vi "Aufschaltung CalGas Span Name.vi"() -> (3 "Span Name":T1)   [LabVIEW 2020, in "Linearisierung v2.lvlib" / "SpanEinstellungen.lvlib"]
uses:
  SpanEinstellungen.lvlib
  Visualisierungs Elemente/String - Eingabefeld.ctl
  Seiten/CalGas Aufschaltung/FGV CalGas Aktionen.ctl
  Sprachverwaltung/FGV Aktion Tabelle zerlegen.ctl
  Seiten/CalGas Aufschaltung/CalGas Aufschaltung.lvlib
  Sprachverwaltung/Sprachverwaltung.lvlib
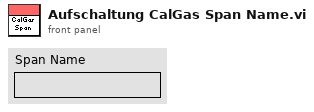
[diagram p1: front panel]
types:
  T1 = typedef "String - Eingabefeld.ctl" = string
  T2 = typedef "Sprachverwaltung.lvlib/FGV Aktion Tabelle zerlegen.ctl" = enum16{"laden", "vereinzeln", "speichern"}
  T3 = typedef "CalGas Aufschaltung.lvlib/FGV CalGas Aktionen.ctl" = enum16{"lesen", "Analysator Auswahl", "Def.CalGas", "Aufschaltung CalGas", "laden", "speichern", "KAL extrahieren"}
  T4 = typedef "CalGas Aufschaltung.lvlib/Aufschaltung CalGas.ctl" = cluster{"Kalibriergas":T5, "Aufschaltpunkt":T6, "Analysator":T7}
  T5 = typedef "Auswahlfeld.ctl" = u16
  T6 = typedef "CalGas Aufschaltung.lvlib/Auswahl Aufschaltpunkt.ctl" = enum16{"über Filterblock", "Analysator direkt", "über PNS", "Entnahme", "Gasdivider"}
  T7 = typedef "CalGas Aufschaltung.lvlib/Auswahl Analysator.ctl" = enum16{"FT-IR", "FID", "PMA", "PMA/FID/FT-IR"}
  T8 = typedef "CalGas Aufschaltung.lvlib/Definition CalGas Anzeige.ctl" = cluster{"Namen":T9, "Werte":T10, "Werte 2":T10, "Einheit":T12, "Messbereiche":T13}
  T9 = typedef "CalGas Aufschaltung.lvlib/CalGas-Namen.ctl" = cluster{"Name":T1, "Name 2":T1, "Name 3":T1, "Name 4":T1, "Name 5":T1, "Name 6":T1, "Name 7":T1, "Name 8":T1, "Name 9":T1, "Name 10":T1, "Name 11":T1, "Name 12":T1}
  T10 = typedef "CalGas Aufschaltung.lvlib/CalGas-Werte.ctl" = cluster{"Konzentration 1":T11, "Konzentration 2":T11, "Konzentration 3":T11, "Konzentration 4":T11, "Konzentration 5":T11, "Konzentration 6":T11, "Konzentration 7":T11, "Konzentration 8":T11, "Konzentration 9":T11, "Konzentration 10":T11, "Konzentration 11":T11, "Konzentration 12":T11}
  T11 = typedef "Zahlen-Eingabefeld.ctl" = sgl
  T12 = typedef "CalGas Aufschaltung.lvlib/CalGas-Einheit.ctl" = cluster{"Einheit 1":T5, "Einheit 2":T5, "Einheit 3":T5, "Einheit 4":T5, "Einheit 5":T5, "Einheit 6":T5, "Einheit 7":T5, "Einheit 8":T5, "Einheit 9":T5, "Einheit 10":T5, "Einheit 11":T5, "Einheit 12":T5}
  T13 = typedef "CalGas Aufschaltung.lvlib/CalGas-Messbereiche.ctl" = cluster{"Messbereich 1":T5, "Messbereich 2":T5, "Messbereich 3":T5, "Messbereich 4":T5, "Messbereich 5":T5, "Messbereich 6":T5, "Messbereich 7":T5, "Messbereich 8":T5, "Messbereich 9":T5, "Messbereich 10":T5, "Messbereich 11":T5, "Messbereich 12":T5}
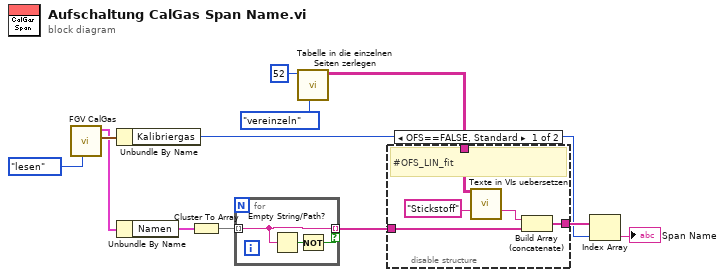
[diagram p0: block diagram]
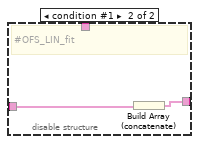
[diagram p2: hidden frame]
diagram:
  n1 = call "FGV CalGas.vi"("Aktionen"=FGV_CalGas_Aktionen."lesen") -> ("Aufschaltung CalGas"=w11:T4, "Def.CalGas"=w8:T8)  [unwired: 6 in, 3 out]
  n2 = Unbundle By Name(w11) -> ("Kalibriergas"=w2:T5)
  n3 = Unbundle By Name(w8) -> ("Namen"=w10:T9)
  n4 = Cluster To Array(cluster=w10) -> (array=w9:T1[])
  n5 = for {
    tunnel: w9 -> [w15] mode=indexing
    tunnel: [w15] -> w7 mode=indexing if=w13
    n6 = Empty String/Path?(string/path=w15) -> (empty?=w14:bool)
    n7 = Not(x=w14) -> (.not. x?=w13:bool)
  }
  n8 = call "Tabelle in die einzelnen Seiten zerlegen.vi"("Aktion"=FGV_Aktion_Tabelle_zerlegen."vereinzeln", "Index (Seite)"=52) -> ("Sprachliste"=w3:string[][])  [unwired: 7 in, 2 out]
  n9 = disable-structure shown="OFS==FALSE, Standard" {
    disable-tunnel: w7 -> [w20 w22]
    disable-tunnel: [w19 w21] -> w6
    disable-tunnel: w3 -> [w18 _]
    frame condition #0 (active) {
      # "#OFS_LIN_fit"
      n10 = call "Texte in VIs uebersetzen.vi"("Sprachliste"=w18, "String zum Übersetzen"="Stickstoff" ("String")) -> ("String zum Übersetzen"=w16:string)  [unwired: 9 in, 4 out]
      n11 = Build Array (concatenate)(w16, w20) -> (w19:T1[])
    }
    frame condition #1 {
      # "#OFS_LIN_fit"
      n12 = Build Array (concatenate)(w22) -> (w21:T1[])
    }
  }
  n13 = Index Array(array=w6, index=w2) -> (element=→"Span Name":T1)
